vi "HOST_feedback+datatrig_AAoptAOD_8-25-23.vi"() -> ()   [LabVIEW 2020]
uses:
  <vilib>/rvi/interface/nirviMethod/nirviMethod.xnode
  <vilib>/rvi/errors/niLvFpgaMergeErrorWithErrorCode.vi
  <instrlib>/_niInstr/Streaming/v1/Host/niInstr Streaming v1 Host.lvlib
  <vilib>/rvi/interface/nirviReadWriteControl/nirviReadWriteControl.xnode
  <vilib>/rvi/interface/nirviCloseFPGA/nirviCloseFPGA.xnode
  <vilib>/rvi/interface/nirviOpenFPGA/nirviOpenFPGA.xnode
  <vilib>/rvi/interface/Simulation/niFpgaSimulationCallBeginRW.vi
  <vilib>/rvi/errors/niLvFpgaAdjustHostInterfaceError.vi
  NiFpgaLv.dll
  <vilib>/Utility/error.llb/Error Cluster From Error Code.vi
  <vilib>/Utility/file.llb/Write Delimited Spreadsheet (string).vi
  <instrlib>/_niInstr/Streaming/v1/Host/Public/Start Finite Stream.vi
  <instrlib>/_niInstr/Streaming/v1/Host/Public/Wait for Stream.vi
  <vilib>/FPGAPlugInAG/Dynamic/niLvFpga_ConfigureFifo_Dynamic.vi
  <vilib>/FPGAPlugInAG/Dynamic/niLvFpga_StartFifo_Dynamic.vi
  <vilib>/FPGAPlugInAG/Dynamic/niLvFpga_ReadFifo_Dynamic.vi
  <vilib>/FPGAPlugInAG/Dynamic/niLvFpga_WriteFifo_Dynamic.vi
  <vilib>/FPGAPlugInAG/Dynamic/niLvFpga_Close_Dynamic.vi
  <vilib>/measure/NI_MAPro.lvlib
  <instrlib>/_niInstr/Streaming/v1/Host/Public/Start Continuous Stream.vi
  FPGA Bitfiles/rfsignal_FPGATarget_feedbackarray+da_BHXJFx-D6v4.lvbitx
  <vilib>/measure/maspectr.llb/FFT Power Spectrum and PSD for N Chan.vi
  <vilib>/FPGAPlugInAG/PXIe-7972R/niLvFpga_Open_PXIe-7972R.vi
  <vilib>/rvi/interface/common/dynamic/niFpgaDynamicAddResources.vi
  <vilib>/userdefined/Silver/nirio_resource_slv.ctl
  Controls/Clock Select.ctl
  PID/Typedef/niFpgaPID_ManualControl.ctl
  PID/Typedef/niFpgaPID_PIDGains.ctl
  PID/Typedef/niFpgaPID_OutputRange.ctl
  PID/Typedef/niFpgaPID_SetpointWeightings.ctl
  PID/Typedef/niFpgaPID_PIDActions.ctl
panel:
  in  "Save data":bool
  in  "File name":string="Z_3mbar_i"
  in  "Save Path Directory":path=path "D:/Lab Data/test"
  out "SUM PSD":cluster{"f0":dbl, "df":dbl, "magnitude":dbl[]}[](graph)
  out "SUM":waveform(dbl)[](graph)=[{"t0"=timestamp(0 s since 1904-01-01), "dt"=0.0002, "Y"=array[1000 elements]}, {"t0"=timestamp(0 s since 1904-01-01), "dt"=0.0002, "Y"=array[1000 elements]}, {"t0"=timestamp(0 s since 1904-01-01), "dt"=0.0002, "Y"=array[1000 elements]}, {"t0"=timestamp(0 s since 1904-01-01), "dt"=0.0002, "Y"=array[1000 elements]}]
  out "Y PSD":cluster{"f0":dbl, "df":dbl, "magnitude":dbl[]}[](graph)
  out "Y":waveform(dbl)[](graph)=[{"t0"=timestamp(0 s since 1904-01-01), "dt"=0.0002, "Y"=array[1000 elements]}, {"t0"=timestamp(0 s since 1904-01-01), "dt"=0.0002, "Y"=array[1000 elements]}, {"t0"=timestamp(0 s since 1904-01-01), "dt"=0.0002, "Y"=array[1000 elements]}, {"t0"=timestamp(0 s since 1904-01-01), "dt"=0.0002, "Y"=array[1000 elements]}]
  out "X PSD":cluster{"f0":dbl, "df":dbl, "magnitude":dbl[]}[](graph)
  out "X":waveform(dbl)[](graph)=[{"t0"=timestamp(0 s since 1904-01-01), "dt"=0.0002, "Y"=array[1000 elements]}, {"t0"=timestamp(0 s since 1904-01-01), "dt"=0.0002, "Y"=array[1000 elements]}, {"t0"=timestamp(0 s since 1904-01-01), "dt"=0.0002, "Y"=array[1000 elements]}, {"t0"=timestamp(0 s since 1904-01-01), "dt"=0.0002, "Y"=array[1000 elements]}]
  in  "Set Point Initialization":bool
  in  "Feedback scaling y":fxp<+,16,4>
  in  "Gains Y":T1[](array[typedef]) {"filter coefficient" min=0 max=1; "proportional gain" step=0.125}
  in  "Gains X":T1[](array[typedef]) {"filter coefficient" min=0 max=1; "proportional gain" step=0.125}
  in  "Data transfer method":bool
  in  "Downsample":i16=1
  in  "Signal Delay (us)":i32=5
  out "actions":T2
  out "error":sgl
  out "output":sgl
  out "error 2":sgl
  out "error 3":sgl
  out "output 3":sgl
  out "actions 3":T2
  out "output 2":sgl
  out "actions 2":T2
  in  "Gains Z":T1[](array[typedef]) {"filter coefficient" min=0 max=1; "proportional gain" step=0.125}
  in  "setpoint weighting 3":T3={"proportional weighting (1)"=1.0, "derivative weighting (0)"=0.0} {"derivative weighting (0)" min=0 max=1; "proportional weighting (1)" min=0 max=1}
  in  "output range 3":T4={"output high (Inf)"=inf, "output low (-Inf)"=-inf}
  in  "manual control 3":T5
  in  "Z reset? (F)":bool
  in  "setpoint weighting 2":T3={"proportional weighting (1)"=1.0, "derivative weighting (0)"=0.0} {"derivative weighting (0)" min=0 max=1; "proportional weighting (1)" min=0 max=1}
  in  "output range 2":T4={"output high (Inf)"=inf, "output low (-Inf)"=-inf}
  in  "manual control 2":T5
  in  "Y reset? (F)":bool
  in  "Feedback scaling z":fxp<+,16,4>
  in  "Feedback scaling x":fxp<+,16,4>
  in  "Apply feedback":bool
  in  "Data Trigger Level (V)":dbl
  in  "Record Size":u32=1024
  out "AI":waveform(dbl)[](graph)
  in  "Data Trigger When":enum8{"Trigger Above", "Trigger Below"}(ring)
  in  "Trigger Type":enum8{"Immediate", "Data Trigger", "TRIG input"}(ring)
  in  "Direction switch":bool
  in  "Step gain values":dbl
  in  "?":bool
  in  "% of max CH 1":dbl=85.0
  in  "% of max CH 0":dbl=90.0
  in  "setpoint weighting":T3={"proportional weighting (1)"=1.0, "derivative weighting (0)"=0.0} {"derivative weighting (0)" min=0 max=1; "proportional weighting (1)" min=0 max=1}
  in  "output range":T4={"output high (Inf)"=inf, "output low (-Inf)"=-inf}
  in  "manual control":T5
  in  "X reset? (F)":bool
  in  "write time ch0":bool
  in  "Record time for power sweep CH0":bool
  in  "Record time for power sweep CH1":bool
  in  "write time ch1":bool
  in  "save path for power calibration (dialog if empty)":path
  out "time check":u16=16
  in  "Cycles per step":u16=30
  in  "Gain Scan Endpoint (CH1)":dbl[](array[numeric])=[100.0, 100.0, 100.0, 100.0, 100.0, 100.0, 100.0, 100.0, 100.0, 100.0, 100.0, 100.0, 100.0, 100.0, 100.0, 100.0, 100.0, 100.0, 100.0, 100.0, 100.0, 100.0, 100.0, 100.0, 100.0, 100.0, 100.0, 100.0, 100.0, 100.0, 100.0, 100.0, 100.0, 100.0, 100.0, 100.0]
  in  "Gain Scan Endpoint (CH0)":dbl[](array[numeric])=[100.0, 100.0, 100.0, 100.0, 100.0, 100.0, 100.0, 100.0, 100.0, 100.0, 100.0, 100.0, 100.0, 100.0, 100.0, 100.0, 100.0, 100.0, 100.0, 100.0, 100.0, 100.0, 100.0, 100.0, 100.0, 100.0, 100.0, 100.0, 100.0, 100.0, 100.0, 100.0, 100.0, 100.0, 100.0, 100.0]
  in  "Scan End Setpoint (CH1)":dbl[](array[numeric])=[23.0, 24.0, 25.0, 26.0, 27.0, 28.0, 23.0, 24.0, 25.0, 26.0, 27.0, 28.0, 23.0, 24.0, 25.0, 26.0, 27.0, 28.0, 23.0, 24.0, 25.0, 26.0, 27.0, 28.0, 23.0, 24.0, 25.0, 26.0, 27.0, 28.0, 23.0, 24.0, 25.0, 26.0, 27.0, 28.0] format="%#_10f"
  in  "Scan CH1":bool
  in  "Scan CH0":bool
  in  "Fq Scan Endpoint (CH0)":dbl[](array[numeric])=[23.0, 23.0, 23.0, 23.0, 23.0, 23.0, 24.0, 24.0, 24.0, 24.0, 24.0, 24.0, 25.0, 25.0, 25.0, 25.0, 25.0, 25.0, 26.0, 26.0, 26.0, 26.0, 26.0, 26.0, 27.0, 27.0, 27.0, 27.0, 27.0, 27.0, 28.0, 28.0, 28.0, 28.0, 28.0, 28.0] format="%#_10f"
  in  "Gain Scan Step Size % (CH1)":dbl=1.0
  in  "Gain Scan Step Size % (CH0)":dbl=1.0
  in  "Fq Scan Step Size MHz (CH1)":dbl=0.1
  in  "Fq Scan Step Size MHz (CH0)":dbl=0.1
  in  "Input pass through\nmode":enum16{"Wire", "Accum-edge"}(ring)=enum."Accum-edge"
  in  "# of beams":u8=36
  in  "Wave Reader CH 1 (MHz)":dbl[](array[numeric])=[23.0, 24.0, 25.0, 26.0, 27.0, 28.0, 23.0, 24.0, 25.0, 26.0, 27.0, 28.0, 23.0, 24.0, 25.0, 26.0, 27.0, 28.0, 23.0, 24.0, 25.0, 26.0, 27.0, 28.0, 23.0, 24.0, 25.0, 26.0, 27.0, 28.0, 23.0, 24.0, 25.0, 26.0, 27.0, 28.0] format="%#_15f"
  in  "Gain CH 1 (%)":dbl[](array[numeric])=[100.0, 100.0, 100.0, 100.0, 100.0, 100.0, 100.0, 100.0, 100.0, 100.0, 100.0, 100.0, 100.0, 100.0, 100.0, 100.0, 100.0, 100.0, 100.0, 100.0, 100.0, 100.0, 100.0, 100.0, 100.0, 100.0, 100.0, 100.0, 100.0, 100.0, 100.0, 100.0, 100.0, 100.0, 100.0, 100.0]
  in  "Remove transition edges":i32=5
  in  "Time per beam in us":i32=20
  in  "stop":bool
  in  "Gain CH 0 (%)":dbl[](array[numeric])=[100.0, 100.0, 100.0, 100.0, 100.0, 100.0, 100.0, 100.0, 100.0, 100.0, 100.0, 100.0, 100.0, 100.0, 100.0, 100.0, 100.0, 100.0, 100.0, 100.0, 100.0, 100.0, 100.0, 100.0, 100.0, 100.0, 100.0, 100.0, 100.0, 100.0, 100.0, 100.0, 100.0, 100.0, 100.0, 100.0]
  in  "Wave Reader CH 0 (MHz)":dbl[](array[numeric])=[23.0, 23.0, 23.0, 23.0, 23.0, 23.0, 24.0, 24.0, 24.0, 24.0, 24.0, 24.0, 25.0, 25.0, 25.0, 25.0, 25.0, 25.0, 26.0, 26.0, 26.0, 26.0, 26.0, 26.0, 27.0, 27.0, 27.0, 27.0, 27.0, 27.0, 28.0, 28.0, 28.0, 28.0, 28.0, 28.0] format="%#_13f"
  in  "Magnitude Initialization Vpp":dbl[](array[numeric])=[1.0, 1.0] format="%0.2p"
  in  "Frequencies (Hz)":dbl[](array[numeric])=[10000.0, 10000.0] format="%5.0p"
  in  "Signal Type":T6(ring)
  in  "Sampling Info":cluster{"Fs":dbl, "#s":dbl}={"Fs"=163840000.0, "#s"=65536.0} {"Fs" format="%#_5p"}
  out "Error Out":errorcluster
  in  "Update Waveform":bool
  in  "Clock Select":T7 items=["Internal Clock", "Internal Clock w/ Ref via CLK/REF IN", "Internal Clock w/ Ref via Sync Clock", "External Clock via CLK/REF IN"]
  in  "Rate of External Sample Clock (MHz)":u16=100 min=60 max=100 step=1
  in  "RIO Resource":T8="RIO0"
  # "Timeshare sampling doesn't work for 1 beam"
  # "General Feedback Settings"
  # "Time cycle loop processing"
  # "up to 65535"
  # "Don't change"
  # "Waveform Initialization"
  # "Controls the Output of the FPGA\nEach row corresponds to one beam created by the AOD\nCH 0 is Output 0 on the FPGA card and controls the () direction on the AOD; CH 1 is Output 1 on the FPGA card and controls the () direction on the AOD\n\nThe  set frequency is the output of the FPGA, this is then mixed with a 50MHz LO to be in the AOD's bandwidth of 75 +- 15MHz\n\nThe gain is the percentage of the 1Vpp initialized voltage to output. It is in percentage and goes from 0 - 100\n\nIt will play the first n rows of tones, \nwhere n is the \"# of beams\" value."
  # "DO NOT CHANGE"
  # "These allow you to smoothly ramp between frequencies or gain settings for each individual beam.\nThe channels scan independently, but it will simultaneously ramp every fq/gain in the channel to their desired point.\nThey should update to match the main control setting when scanning is not enabled."
  # "X Feedback"
  # "Do not change these values while waiting for scan"
  # "Main control for the tones played on FPGA analog out 0\nSets the base, static frequency to play"
  # "Main control for the tones played on FPGA analog out 1\nSets the base, static frequency to play"
  # "Ch 0 Output Waveforms"
  # "Ch 1 Output Waveforms"
  # "Y Feedback"
  # "Ch0"
  # "Ch1"
  # "Z Feedback"
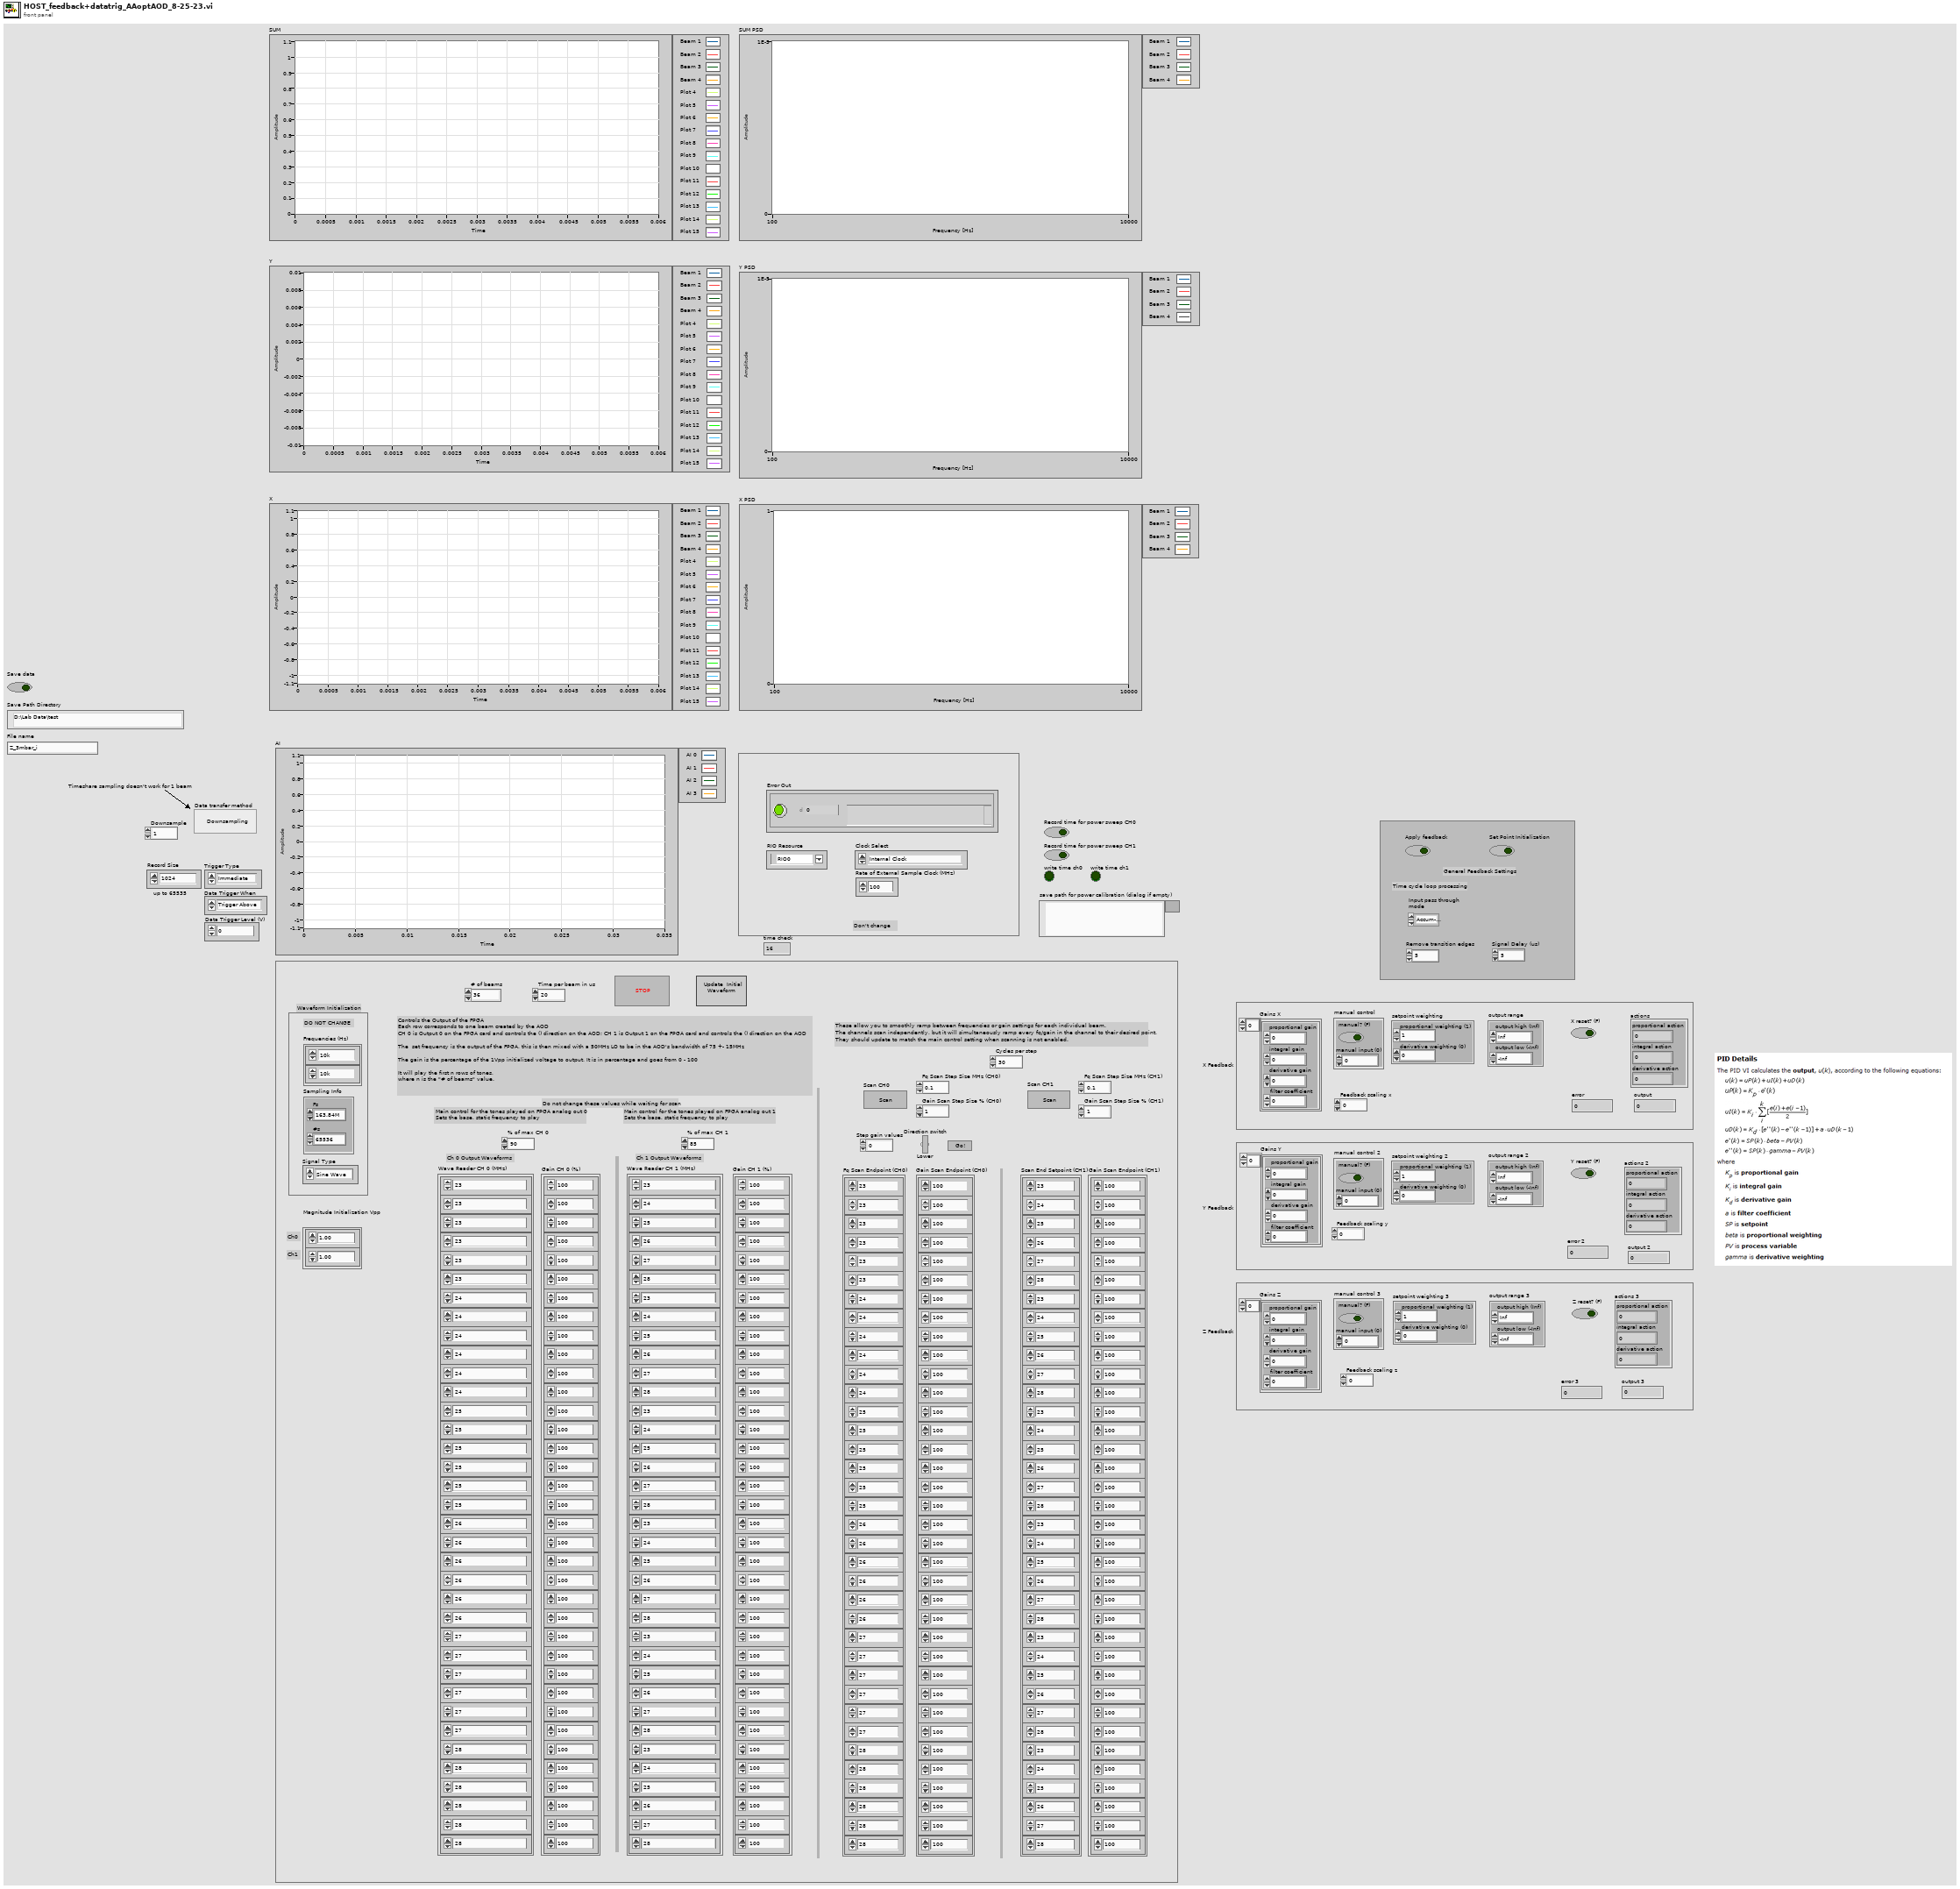
[diagram p1: front panel]
types:
  T1 = typedef "niFpgaPID_PIDGains.ctl" = cluster{"proportional gain":sgl, "integral gain":sgl, "derivative gain":sgl, "filter coefficient":sgl}
  T2 = typedef "niFpgaPID_PIDActions.ctl" = cluster{"proportional action":sgl, "integral action":sgl, "derivative action":sgl}
  T3 = typedef "niFpgaPID_SetpointWeightings.ctl" = cluster{"proportional weighting (1)":sgl, "derivative weighting (0)":sgl}
  T4 = typedef "niFpgaPID_OutputRange.ctl" = cluster{"output high (Inf)":sgl, "output low (-Inf)":sgl}
  T5 = typedef "niFpgaPID_ManualControl.ctl" = cluster{"manual? (F)":bool, "manual input (0)":sgl}
  T6 = enum16{"Sine Wave", "Triangle Wave", "Square Wave", "Sawtooth Wave"}
  T7 = typedef "Clock Select.ctl" = u16
  T8 = typedef "nirio_resource_slv.ctl" = tag
  T9 = cluster{"proportional action":sgl, "integral action":sgl, "derivative action":sgl}
  T10 = cluster{"level":i16, "trigger when":enum8{"Trigger Above", "Trigger Below"}}
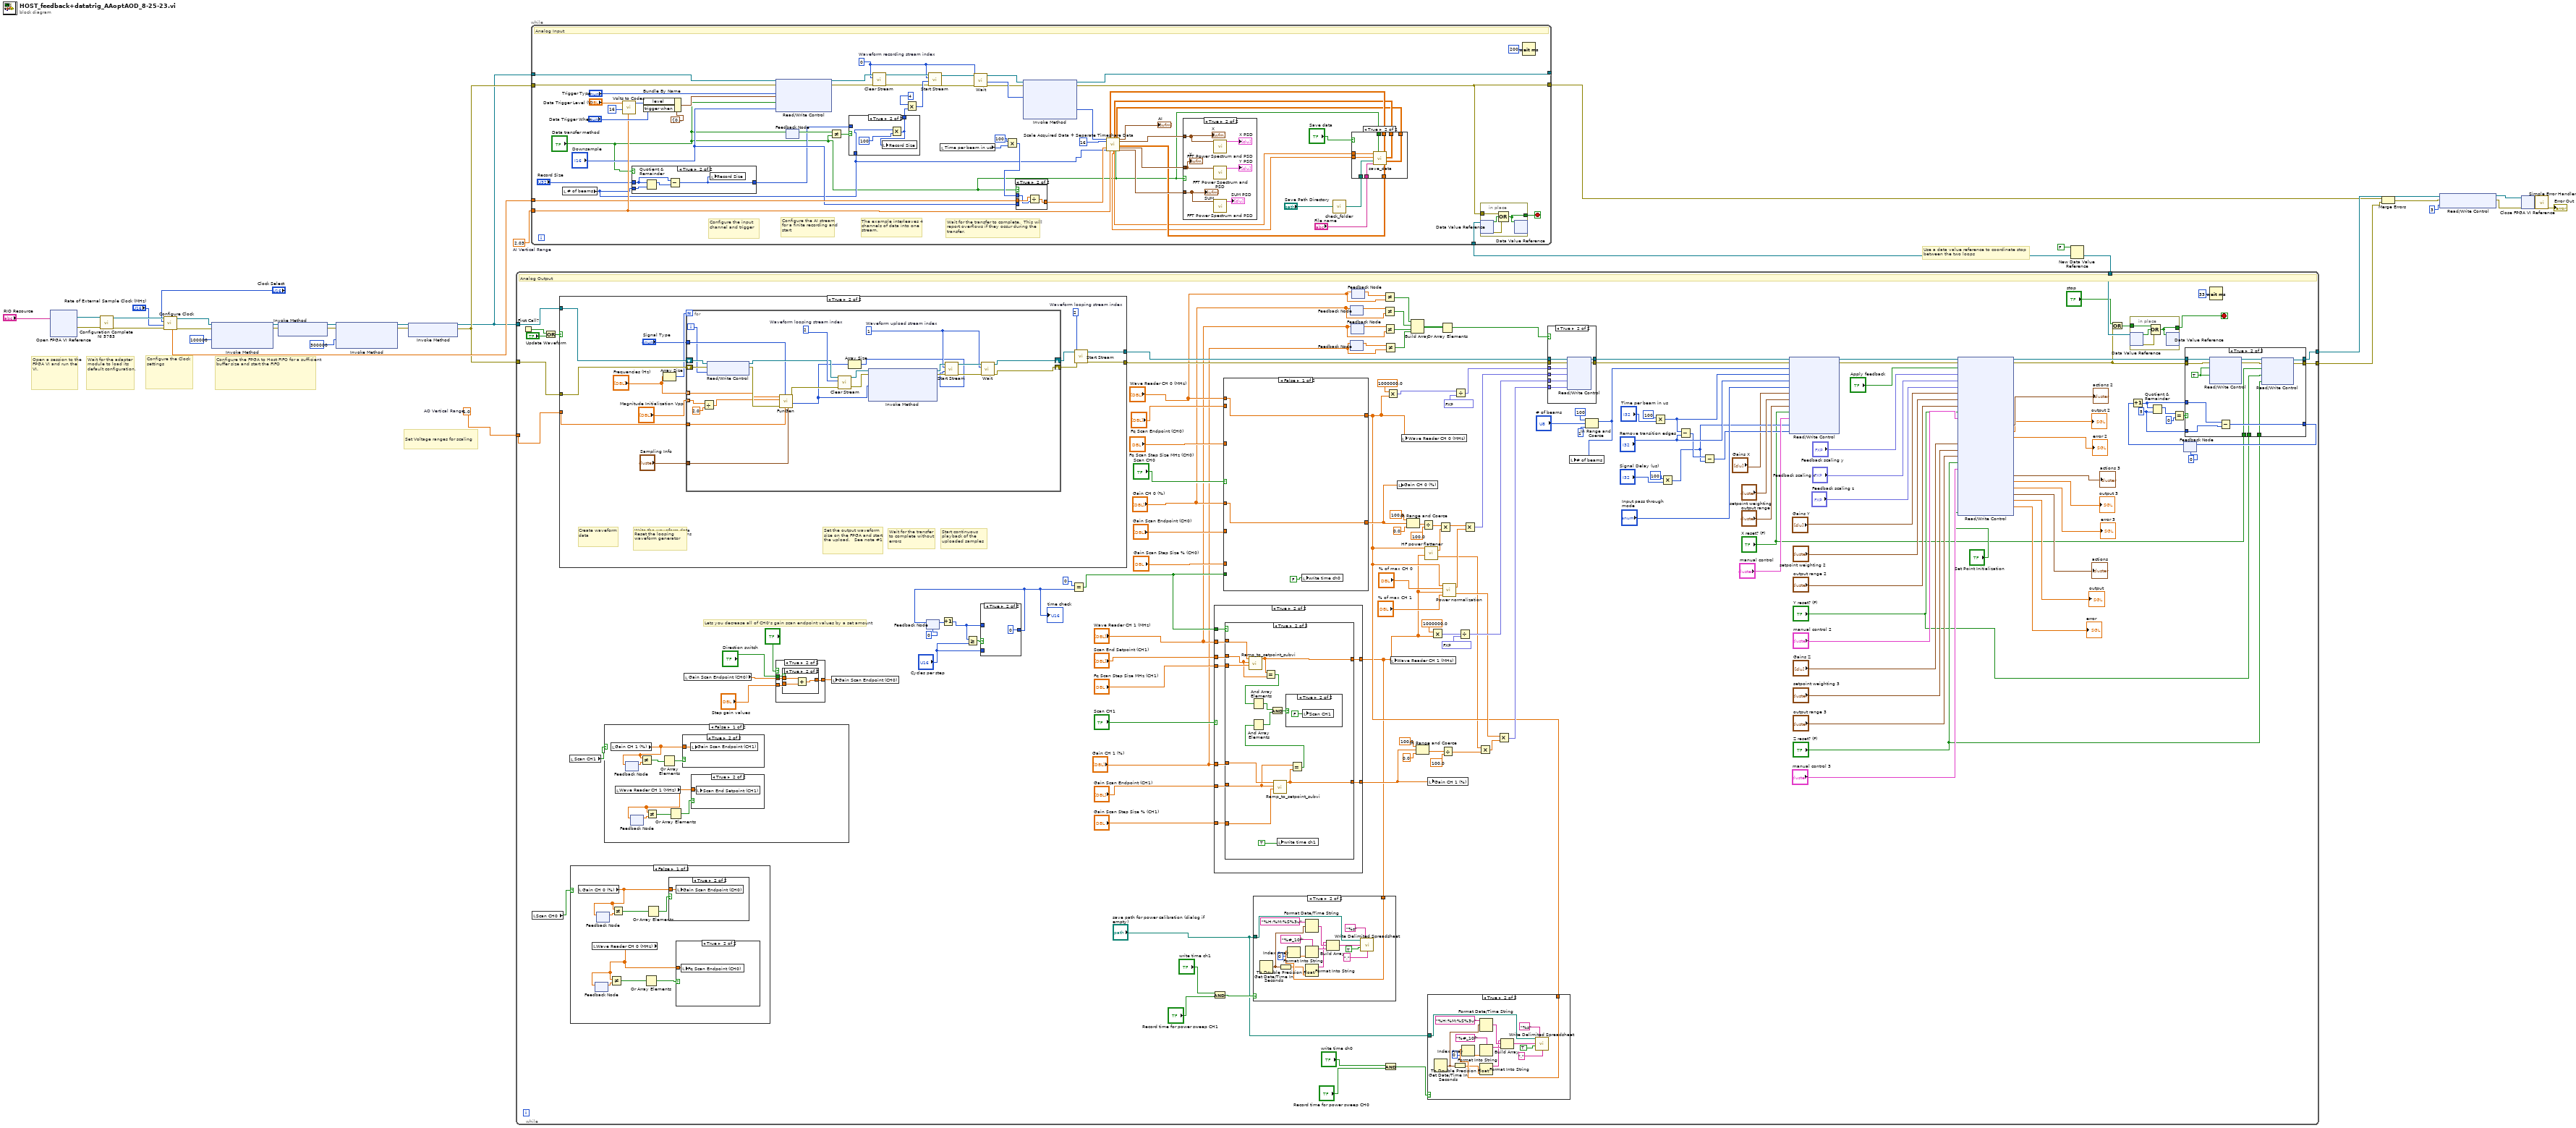
[diagram p0: block diagram]
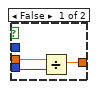
[diagram p6: hidden frame]
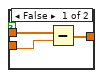
[diagram p10: hidden frame]
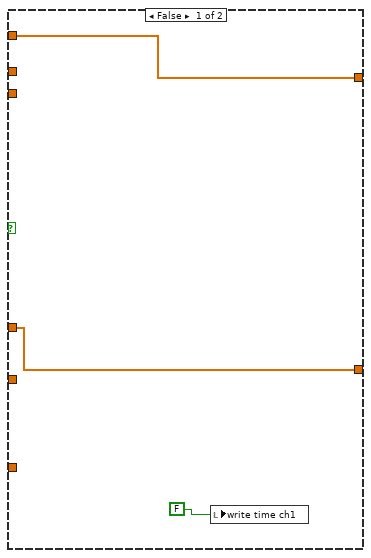
[diagram p13: hidden frame]
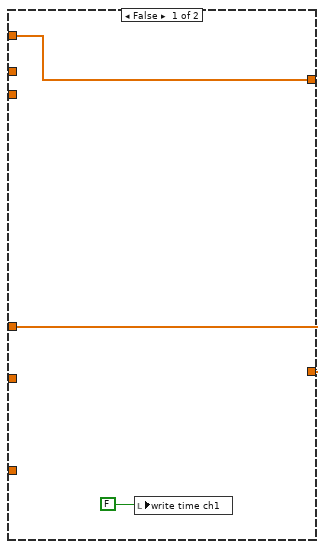
[diagram p14: hidden frame]
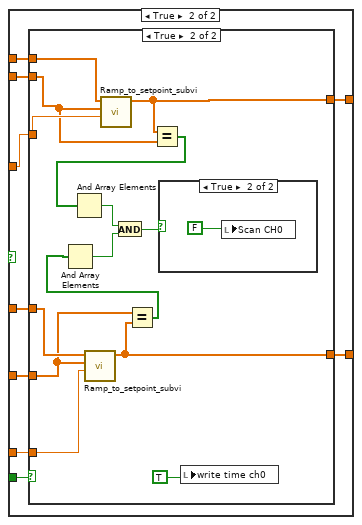
[diagram p16: hidden frame]
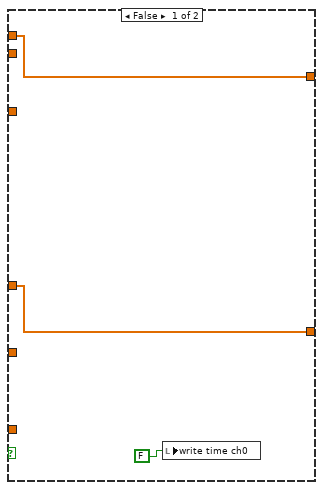
[diagram p17: hidden frame]
diagram:
  w13 = 2.03  # AI Vertical Range
  w21 = 1.0  # AO Vertical Range
  # "Use a data value reference to coordinate stop between the two loops"
  # "Set Voltage ranges for scaling"
  # "Configure the Clock settings"
  # "Configure the FPGA to Host FIFO for a sufficient buffer size and start the FIFO"
  # "Wait for the adapter module to load its default configuration."
  # "Open a session to the FPGA VI and run the VI."
  n1 = xnode "Open FPGA VI Reference"("resource name"="RIO Resource") -> ("FPGA VI Reference Out"=w19:refnum<k20>, "error out"=w18:errorcluster)  [unwired: 1 in]
  n2 = call "Configuration Complete NI 5783.vi"("error in"=w18, "FPGA VI Reference In"=w19) -> ("error out"=w29:errorcluster, "FPGA VI Reference Out"=w30:refnum<k20>)  [unwired: 7 in, 1 out]
  n3 = call "Configure Clock.vi"("error in (no error)"=w29, "Rate of External Sample Clock (MHz)"="Rate of External Sample Clock (MHz)", "Clock Select"="Clock Select", "FPGA VI Reference In"=w30) -> ("error out"=w27:errorcluster, "FPGA VI Reference Out"=w28:refnum<k20>, "Sampling Rate"=w12:dbl)  [unwired: 3 in, 2 out]
  n4 = xnode "Invoke Method"("FPGA VI Reference In"=w28, "error in"=w27, "Requested Depth"=u32 100000) -> ("FPGA VI Reference Out"=w33:refnum<k20>, "error out"=w32:errorcluster)  [unwired: 1 out]
  n5 = xnode "Invoke Method"("FPGA VI Reference In"=w33, "error in"=w32) -> ("FPGA VI Reference Out"=w5:refnum<k20>, "error out"=w8:errorcluster)
  n6 = xnode "Invoke Method"("FPGA VI Reference In"=w5, "error in"=w8, "Requested Depth"=u32 300000) -> ("FPGA VI Reference Out"=w4:refnum<k20>, "error out"=w7:errorcluster)  [unwired: 1 out]
  n7 = xnode "Invoke Method"("FPGA VI Reference In"=w4, "error in"=w7) -> ("FPGA VI Reference Out"=w3:refnum<k20>, "error out"=w6:errorcluster)
  n8 = New Data Value Reference(data value=FALSE ("Stopped")) -> (data value reference=w1:refnum<data-value>)  [unwired: 1 in, 1 out]
  n9 = while {
    tunnel: w6 -> [w177]
    tunnel: w3 -> [w183]
    tunnel: [w39] -> w17
    tunnel: w1 -> [w178]
    tunnel: w21 -> [w176]
    tunnel: [w38] -> w9
    stop <- w108 stop-if-true
    w41 = 5
    # "Lets you decrease all of CH0's gain scan endpoint values by a set amount"
    # "Analog Output"
    n10 = First Call?() -> (First Call?: T/F=w179:bool)
    n11 = local read "Scan CH0"() -> (w146:bool)
    n12 = Or(x=w179, y="Update Waveform") -> (x .or. y?=w180:bool)
    n13 = case shown="True" w180 {
      tunnel: [w338 w351] -> w175
      tunnel: [w337 w350] -> w174
      tunnel: w183 -> [w338 w348]
      tunnel: w177 -> [w337 w347]
      tunnel: w176 -> [_ w349]
      frame False {
      }
      frame True {
        w346 = 2  # Waveform looping stream index
        # "Loop over the waveforms to combine"
        # "Reset the looping waveform generator"
        # "Start continuous playback of the uploaded samples"
        # "Wait for the transfer to complete without errors"
        # "Set the output waveform size on the FPGA and start the upload.   See note #1"
        # "Write the waveform data to the FPGA for generation"
        # "Create waveform data"
        n14 = Array Size(array="Frequencies (Hz)") -> (size(s)=w341:i32)
        n15 = for {
          N: w341 -> [_]
          tunnel: w349 -> [w366]
          shift-right: [w360] -> w345
          shift-left: w348 -> [w365]
          shift-right: [w359] -> w344
          shift-left: w347 -> [w363]
          tunnel: "Frequencies (Hz)" -> [w358] mode=indexing
          tunnel: "Magnitude Initialization Vpp" -> [w354] mode=indexing
          tunnel: "Sampling Info" -> [w357]
          tunnel: "Signal Type" -> [w356]
          i -> [w355]
          w367 = 2  # Waveform looping stream index
          w372 = 1  # Waveform upload stream index
          n16 = Divide(x=w354, y=2.0) -> (x/y=w353:dbl)
          n17 = xnode "Read/Write Control"("FPGA VI Reference In"=w365, "error in"=w363, "Upload selector"=w355) -> ("FPGA VI Reference Out"=w364:refnum<k20>, "error out"=w362:errorcluster)
          n18 = call "FunGen.vi"("sampling info"=w357, "range (Vpp)"=w366, "signal type"=w356, "error in (no error)"=w362, "amplitude"=w353, "frequency"=w358) -> ("error out"=w368:errorcluster, "Waveform Data"=w361:i16[])  [unwired: 2 in, 2 out]
          n19 = call <instrlib>:"Clear Stream.vi"("error in (no error)"=w368, "stream index"=w367, "refnum in"=w364) -> ("error out"=w370:errorcluster, "refnum out"=w371:refnum<k20>)  [unwired: 7 in]
          n20 = Array Size(array=w361) -> (size(s)=w369:i32)
          n21 = xnode "Invoke Method"("FPGA VI Reference In"=w371, "error in"=w370, "Data"=w361) -> ("FPGA VI Reference Out"=w376:refnum<k20>, "error out"=w375:errorcluster)  [unwired: 1 in, 1 out]
          n22 = call-poly <instrlib>:"Start Stream.vi"("error in (no error)"=w375, "num samples"=w369, "stream index"=w372, "refnum in"=w376) -> ("error out"=w373:errorcluster, "refnum out"=w374:refnum<k20>)  [unwired: 6 in]
          n23 = call-poly <instrlib>:"Wait.vi"("error in (no error)"=w373, "stream index"=w372, "refnum in"=w374) -> ("error out"=w359:errorcluster, "refnum out"=w360:refnum<k20>)  [unwired: 5 in, 2 out]
        }
        n24 = call-poly <instrlib>:"Start Stream.vi"("error in (no error)"=w344, "stream index"=w346, "refnum in"=w345) -> ("error out"=w350:errorcluster, "refnum out"=w351:refnum<k20>)  [unwired: 7 in]
      }
    }
    n25 = local read "Scan CH1"() -> (w147:bool)
    n26 = case shown="False" w146 {
      frame False {
        n27 = local read "Gain CH 0 (%)"() -> (w313:dbl[])
        n28 = local read "Wave Reader CH 0 (MHz)"() -> (w320:dbl[])
        n29 = feedback-in #1(w320) -> ()
        n30 = feedback #1() -> (w319:dbl[])  [unwired: 1 in]
        n31 = feedback #2() -> (w316:dbl[])  [unwired: 1 in]
        n32 = feedback-in #2(w313) -> ()
        n33 = Not Equal?(x=w320, y=w319) -> (x != y?=w318:bool[])
        n34 = Not Equal?(x=w313, y=w316) -> (x != y?=w315:bool[])
        n35 = Or Array Elements(Boolean array=w318) -> (logical OR=w317:bool)
        n36 = Or Array Elements(Boolean array=w315) -> (logical OR=w314:bool)
        n37 = case shown="True" w314 {
          tunnel: w313 -> [_ w321]
          frame False {
          }
          frame True {
            n38 = local write "Gain Scan Endpoint (CH0)"(w321) -> ()
          }
        }
        n39 = case shown="True" w317 {
          tunnel: w320 -> [_ w322]
          frame False {
          }
          frame True {
            n40 = local write "Fq Scan Endpoint (CH0)"(w322) -> ()
          }
        }
      }
      frame True {
      }
    }
    n41 = case shown="False" w147 {
      frame False {
        n42 = local read "Gain CH 1 (%)"() -> (w323:dbl[])
        n43 = local read "Wave Reader CH 1 (MHz)"() -> (w327:dbl[])
        n44 = feedback #3() -> (w326:dbl[])  [unwired: 1 in]
        n45 = feedback-in #3(w323) -> ()
        n46 = feedback #4() -> (w330:dbl[])  [unwired: 1 in]
        n47 = feedback-in #4(w327) -> ()
        n48 = Not Equal?(x=w323, y=w326) -> (x != y?=w325:bool[])
        n49 = Not Equal?(x=w327, y=w330) -> (x != y?=w329:bool[])
        n50 = Or Array Elements(Boolean array=w325) -> (logical OR=w324:bool)
        n51 = Or Array Elements(Boolean array=w329) -> (logical OR=w328:bool)
        n52 = case shown="True" w324 {
          tunnel: w323 -> [_ w331]
          frame False {
          }
          frame True {
            n53 = local write "Gain Scan Endpoint (CH1)"(w331) -> ()
          }
        }
        n54 = case shown="True" w328 {
          tunnel: w327 -> [_ w332]
          frame False {
          }
          frame True {
            n55 = local write "Scan End Setpoint (CH1)"(w332) -> ()
          }
        }
      }
      frame True {
      }
    }
    n56 = local read "Gain Scan Endpoint (CH0)"() -> (w110:dbl[])
    n57 = case shown="True" "?" {
      tunnel: w110 -> [w210 w213]
      tunnel: [w210 w214] -> w111
      tunnel: "Step gain values" -> [_ w212]
      tunnel: "Direction switch" -> [_ w211]
      frame False {
      }
      frame True {
        n58 = case shown="True" w211 {
          tunnel: [w217 w219] -> w214
          tunnel: w213 -> [w216 w218]
          tunnel: w212 -> [w215 w220]
          frame False {
            n59 = Subtract(x=w216, y=w215) -> (x-y=w217:dbl[])
          }
          frame True {
            n60 = Add(x=w218, y=w220) -> (x+y=w219:dbl[])
          }
        }
      }
    }
    n61 = local write "Gain Scan Endpoint (CH0)"(w111) -> ()
    n62 = feedback #5(u16 0) -> (w142:u16)
    n63 = Increment(x=w142) -> (x+1=w140:u16)
    n64 = Greater Or Equal?(x=w140, y="Cycles per step") -> (x >= y?=w141:bool)
    n65 = case shown="True" w141 {
      tunnel: w140 -> [w311 _]
      tunnel: "Cycles per step" -> [_ _]
      tunnel: [w311 u16 0] -> w135
      frame False {
      }
      frame True {
      }
    }
    "time check" <- w135
    n66 = feedback-in #5(w135) -> ()
    n67 = Equal?(x=u16 0, y=w135) -> (x = y?=w136:bool)
    n68 = And(x="write time ch1", y="Record time for power sweep CH1") -> (x .and. y?=w134:bool)
    n69 = case shown="True" "Scan CH1" {
      tunnel: "Fq Scan Step Size MHz (CH1)" -> [_ w262]
      tunnel: [w253 w261] -> w70
      tunnel: "Wave Reader CH 1 (MHz)" -> [w253 w260]
      tunnel: "Scan End Setpoint (CH1)" -> [_ w259]
      tunnel: "Gain Scan Step Size % (CH1)" -> [_ w258]
      tunnel: "Gain CH 1 (%)" -> [w252 w257]
      tunnel: "Gain Scan Endpoint (CH1)" -> [_ w256]
      tunnel: [w252 w255] -> w148
      tunnel: w136 -> [_ w254]
      frame False {
        n70 = local write "write time ch1"(FALSE) -> ()
      }
      frame True {
        n71 = case shown="True" w254 {
          tunnel: w260 -> [w265 w279]
          tunnel: w259 -> [_ w277]
          tunnel: w262 -> [_ w278]
          tunnel: [w265 w276] -> w261
          tunnel: w257 -> [w264 w274]
          tunnel: w256 -> [_ w273]
          tunnel: w258 -> [_ w272]
          tunnel: [w264 w267] -> w255
          frame False {
            n72 = local write "write time ch1"(FALSE) -> ()
          }
          frame True {
            n73 = call "Ramp_to_setpoint_subvi.vi"("Numeric"=w278, "Scan to Fq (CH0)"=w277, "Wave Reader CH 0 (Y)"=w279) -> ("Array"=w276:dbl[])  [unwired: 8 in]
            n74 = Equal?(x=w276, y=w277) -> (x = y?=w275:bool[])
            n75 = And Array Elements(Boolean array=w275) -> (logical AND=w269:bool)
            n76 = call "Ramp_to_setpoint_subvi.vi"("Numeric"=w272, "Scan to Fq (CH0)"=w273, "Wave Reader CH 0 (Y)"=w274) -> ("Array"=w267:dbl[])  [unwired: 8 in]
            n77 = local write "write time ch1"(TRUE) -> ()
            n78 = Equal?(x=w273, y=w267) -> (x = y?=w268:bool[])
            n79 = And Array Elements(Boolean array=w268) -> (logical AND=w270:bool)
            n80 = And(x=w269, y=w270) -> (x .and. y?=w271:bool)
            n81 = case shown="True" w271 {
              frame False {
              }
              frame True {
                n82 = local write "Scan CH1"(FALSE) -> ()
              }
            }
          }
        }
      }
    }
    n83 = case shown="False" "Scan CH0" {
      tunnel: "Fq Scan Step Size MHz (CH0)" -> [_ w292]
      tunnel: "Wave Reader CH 0 (MHz)" -> [w283 w291]
      tunnel: "Fq Scan Endpoint (CH0)" -> [_ w290]
      tunnel: [w283 w289] -> w73
      tunnel: "Gain CH 0 (%)" -> [w282 w288]
      tunnel: "Gain Scan Endpoint (CH0)" -> [_ w287]
      tunnel: [w282 w286] -> w155
      tunnel: "Gain Scan Step Size % (CH0)" -> [_ w285]
      tunnel: w136 -> [_ w284]
      frame False {
        n84 = local write "write time ch0"(FALSE) -> ()
      }
      frame True {
        n85 = case shown="True" w284 {
          tunnel: w291 -> [w295 w309]
          tunnel: w290 -> [_ w307]
          tunnel: w292 -> [_ w308]
          tunnel: [w295 w306] -> w289
          tunnel: w288 -> [w294 w304]
          tunnel: w287 -> [_ w301]
          tunnel: w285 -> [_ w303]
          tunnel: [w294 w302] -> w286
          frame False {
            n86 = local write "write time ch0"(FALSE) -> ()
          }
          frame True {
            n87 = call "Ramp_to_setpoint_subvi.vi"("Numeric"=w303, "Scan to Fq (CH0)"=w301, "Wave Reader CH 0 (Y)"=w304) -> ("Array"=w302:dbl[])  [unwired: 8 in]
            n88 = call "Ramp_to_setpoint_subvi.vi"("Numeric"=w308, "Scan to Fq (CH0)"=w307, "Wave Reader CH 0 (Y)"=w309) -> ("Array"=w306:dbl[])  [unwired: 8 in]
            n89 = Equal?(x=w301, y=w302) -> (x = y?=w300:bool[])
            n90 = And Array Elements(Boolean array=w300) -> (logical AND=w297:bool)
            n91 = Equal?(x=w306, y=w307) -> (x = y?=w305:bool[])
            n92 = And Array Elements(Boolean array=w305) -> (logical AND=w298:bool)
            n93 = And(x=w298, y=w297) -> (x .and. y?=w299:bool)
            n94 = case shown="True" w299 {
              frame False {
              }
              frame True {
                n95 = local write "Scan CH0"(FALSE) -> ()
              }
            }
            n96 = local write "write time ch0"(TRUE) -> ()
          }
        }
      }
    }
    n97 = case shown="True" w134 {
      tunnel: w70 -> [_ w243]
      tunnel: "save path for power calibration (dialog if empty)" -> [_ w236]
      frame False {
      }
      frame True {
        n98 = Get Date/Time In Seconds() -> (seconds since 1Jan1904=w239:timestamp)
        n99 = To Double Precision Float(number=w239) -> (double precision float=w238:dbl)
        n100 = Index Array(array=w243, index=0) -> (element=w241:dbl)
        n101 = Format Date/Time String(time format string (%c)="%H:%M:%S%3u", seconds (now)=w239) -> (date/time string=w246:string)  [unwired: 1 in]
        n102 = Format Into String(format string="%#_10f", w241) -> (resulting string=w245:string)  [unwired: 2 in, 1 out]
        n103 = Format Into String(w238) -> (resulting string=w237:string)  [unwired: 3 in, 1 out]
        n104 = Build Array(w237, w246, w245) -> (w240:string[])
        n105 = call-poly <vilib>:"Write Delimited Spreadsheet.vi"("file path (dialog if empty)"=w236, "format (%s)"="%s" ("format (%.3f)"), "1D data"=w240, "append to file? (new file:F)"=TRUE, "delimiter (\\t)"="," ("delimiter (\\t)")) -> ()  [unwired: 9 in, 2 out]
      }
    }
    n106 = feedback-in #6("Gain CH 0 (%)") -> ()
    n107 = feedback #6() -> (w64:dbl[])  [unwired: 1 in]
    n108 = feedback #7() -> (w60:dbl[])  [unwired: 1 in]
    n109 = feedback-in #7("Gain CH 1 (%)") -> ()
    n110 = feedback #8() -> (w62:dbl[])  [unwired: 1 in]
    n111 = feedback-in #8("Wave Reader CH 1 (MHz)") -> ()
    n112 = feedback #9() -> (w65:dbl[])  [unwired: 1 in]
    n113 = feedback-in #9("Wave Reader CH 0 (MHz)") -> ()
    n114 = Not Equal?(x=w65, y="Wave Reader CH 0 (MHz)") -> (x != y?=w58:bool[])
    n115 = Not Equal?(x=w64, y="Gain CH 0 (%)") -> (x != y?=w57:bool[])
    n116 = Not Equal?(x=w62, y="Wave Reader CH 1 (MHz)") -> (x != y?=w56:bool[])
    n117 = Not Equal?(x=w60, y="Gain CH 1 (%)") -> (x != y?=w55:bool[])
    n118 = And(x="write time ch0", y="Record time for power sweep CH0") -> (x .and. y?=w130:bool)
    n119 = Multiply(x=1000000.0, y=w73) -> (x*y=w164:fxp<+/-,64,32>[])
    n120 = local write "Wave Reader CH 1 (MHz)"(w70) -> ()
    n121 = local write "Gain CH 0 (%)"(w155) -> ()
    n122 = local write "Wave Reader CH 0 (MHz)"(w73) -> ()
    n123 = In Range and Coerce(upper limit=100.0, x=w155, lower limit=0.0) -> (coerced(x)=w158:dbl[])  [unwired: 1 out]
    n124 = Build Array(w58, w57, w56, w55) -> (w54:bool[][])
    n125 = In Range and Coerce(upper limit=100.0, x=w148, lower limit=0.0) -> (coerced(x)=w153:dbl[])  [unwired: 1 out]
    n126 = Divide(x=w158, y=100.0) -> (x/y=w121:dbl[])
    n127 = call "HF power flattener.vi"("CH 1 frequency"=w70, "CH 0 frequency"=w73) -> ("Normalized CH1"=w67:dbl[], "Normalized CH 0"=w71:dbl[])  [unwired: 2 in]
    n128 = local write "Gain CH 1 (%)"(w148) -> ()
    n129 = case shown="True" w130 {
      tunnel: w73 -> [_ w228]
      tunnel: "save path for power calibration (dialog if empty)" -> [_ w221]
      frame False {
      }
      frame True {
        n130 = Get Date/Time In Seconds() -> (seconds since 1Jan1904=w224:timestamp)
        n131 = To Double Precision Float(number=w224) -> (double precision float=w223:dbl)
        n132 = Index Array(array=w228, index=0) -> (element=w226:dbl)
        n133 = Format Date/Time String(time format string (%c)="%H:%M:%S%3u", seconds (now)=w224) -> (date/time string=w231:string)  [unwired: 1 in]
        n134 = Format Into String(format string="%#_10f", w226) -> (resulting string=w230:string)  [unwired: 2 in, 1 out]
        n135 = Format Into String(w223) -> (resulting string=w222:string)  [unwired: 3 in, 1 out]
        n136 = Build Array(w222, w231, w230) -> (w225:string[])
        n137 = call-poly <vilib>:"Write Delimited Spreadsheet.vi"("file path (dialog if empty)"=w221, "format (%s)"="%s" ("format (%.3f)"), "1D data"=w225, "append to file? (new file:F)"=TRUE, "delimiter (\\t)"="," ("delimiter (\\t)")) -> ()  [unwired: 9 in, 2 out]
      }
    }
    n138 = Multiply(x=1000000.0, y=w70) -> (x*y=w162:fxp<+/-,64,32>[])
    n139 = Multiply(x=w121, y=w71) -> (x*y=w72:dbl[])
    n140 = Or Array Elements(Boolean array=w54) -> (logical OR=w53:bool)
    n141 = Divide(x=w153, y=100.0) -> (x/y=w68:dbl[])
    n142 = call "Power normalization.vi"("% of max CH 1"="% of max CH 1", "CH 1 frequency"=w70, "% of max CH 0"="% of max CH 0", "CH 0 frequency"=w73) -> ("Normalized CH1"=w116:dbl[], "Normalized CH 0"=w118:dbl[])
    n143 = Divide(x=w164, y=fxp<+,32,16> 6103.515625) -> (x/y=w127:fxp<+,33,16>[])
    n144 = Divide(x=w162, y=fxp<+,32,16> 6103.515625) -> (x/y=w126:fxp<+,33,16>[])
    n145 = Multiply(x=w72, y=w118) -> (x*y=w122:fxp<+,32,4>[])
    n146 = Multiply(x=w67, y=w68) -> (x*y=w69:dbl[])
    n147 = Multiply(x=w116, y=w69) -> (x*y=w117:fxp<+,32,4>[])
    n148 = case shown="True" w53 {
      tunnel: w175 -> [w201 w209]
      tunnel: w174 -> [w200 w208]
      tunnel: [w201 w207] -> w172
      tunnel: [w200 w206] -> w171
      tunnel: w127 -> [_ w205]
      tunnel: w126 -> [_ w204]
      tunnel: w122 -> [_ w203]
      tunnel: w117 -> [_ w202]
      frame False {
      }
      frame True {
        n149 = xnode "Read/Write Control"("FPGA VI Reference In"=w209, "error in"=w208, "Wave 1"=w205, "Amp 1"=w203, "Wave 2"=w204, "Amp 2"=w202) -> ("FPGA VI Reference Out"=w207:refnum<k20>, "error out"=w206:errorcluster)
      }
    }
    n150 = In Range and Coerce(upper limit=u8 100, x="# of beams", lower limit=u8 1) -> (coerced(x)=w49:u8)  [unwired: 1 out]
    n151 = local write "# of beams"(w49) -> ()
    n152 = Multiply(x=100, y="Time per beam in us") -> (x*y=w85:i32)
    n153 = Multiply(x=100, y="Signal Delay (us)") -> (x*y=w82:i32)
    n154 = Subtract(x=w85, y="Remove transition edges") -> (x-y=w83:i32)
    n155 = Subtract(x=w83, y=w82) -> (x-y=w81:i32)
    n156 = xnode "Read/Write Control"("FPGA VI Reference In"=w172, "error in"=w171, "Size"=w49, "Timeshare"=w85, "Edge size"="Remove transition edges", "Pass selector"="Input pass through\nmode", "Gains X"="Gains X", "setpoint weighting"="setpoint weighting", "output range"="output range", "X reset? (F)"="X reset? (F)", "manual control"="manual control", "Signal Delay"=w82, "Data collection size"=w81) -> ("FPGA VI Reference Out"=w104:refnum<k20>, "error out"=w105:errorcluster)
    n157 = xnode "Read/Write Control"("FPGA VI Reference In"=w104, "error in"=w105, "Apply feedback"="Apply feedback", "Feedback scaling y"="Feedback scaling y", "Feedback scaling x"="Feedback scaling x", "Feedback scaling z"="Feedback scaling z", "Gains Y"="Gains Y", "setpoint weighting 2"="setpoint weighting 2", "output range 2"="output range 2", "Y reset? (F)"="Y reset? (F)", "manual control 2"="manual control 2", "Gains Z"="Gains Z", "setpoint weighting 3"="setpoint weighting 3", "output range 3"="output range 3", "Z reset? (F)"="Z reset? (F)", "manual control 3"="manual control 3", "Set Point Initialization"="Set Point Initialization") -> ("FPGA VI Reference Out"=w40:refnum<k20>, "error out"=w37:errorcluster, "actions 2"=→"actions 2":T9, "output 2"=→"output 2":sgl, "error 2"=→"error 2":sgl, "actions 3"=→"actions 3":T9, "output 3"=→"output 3":sgl, "error 3"=→"error 3":sgl, "actions"=→"actions":T9, "output"=→"output":sgl, "error"=→"error":sgl)
    n158 = Or(x="stop", y=w37) -> (x .or. y?=w107:bool)
    n159 = in-place {
      in-place-border: [w335] -> w108
      in-place-border: w107 -> [w333]
      n160 = in-place-dvr #10(w178) -> (w336:bool, w334:errorcluster)
      n161 = Compound Arithmetic op=OR(w333, w336, w334) -> (w335:bool)
      n162 = in-place-dvr #10(w335) -> ()  [unwired: 2 out]
    }
    n163 = feedback #11(0) -> (w47:i32)
    n164 = Increment(x=w47) -> (x+1=w45:i32)
    n165 = Quotient & Remainder(x=w45, y=w41) -> (x-y*floor(x/y)=w43:i32)  [unwired: 1 out]
    n166 = Equal?(x=w43, y=0) -> (x = y?=w44:bool)
    n167 = case shown="True" w44 {
      tunnel: [w184 w198] -> w48
      tunnel: w45 -> [w184 w199]
      tunnel: w41 -> [_ w197]
      tunnel: w40 -> [w186 w196]
      tunnel: [w186 w190] -> w39
      tunnel: [w185 w191] -> w38
      tunnel: w37 -> [w185 w195]
      tunnel: "Z reset? (F)" -> [_ w189]
      tunnel: "Y reset? (F)" -> [_ w188]
      tunnel: "X reset? (F)" -> [_ w187]
      frame False {
      }
      frame True {
        w194 = TRUE
        n168 = xnode "Read/Write Control"("FPGA VI Reference In"=w196, "error in"=w195, "X reset? (F)"=w194, "Y reset? (F)"=w194, "Z reset? (F)"=w194) -> ("FPGA VI Reference Out"=w193:refnum<k20>, "error out"=w192:errorcluster)
        n169 = Subtract(x=w199, y=w197) -> (x-y=w198:i32)
        n170 = xnode "Read/Write Control"("FPGA VI Reference In"=w193, "error in"=w192, "X reset? (F)"=w187, "Y reset? (F)"=w188, "Z reset? (F)"=w189) -> ("FPGA VI Reference Out"=w190:refnum<k20>, "error out"=w191:errorcluster)
      }
    }
    n171 = feedback-in #11(w48) -> ()
    n172 = Wait (ms)(milliseconds to wait=u32 33) -> ()  [unwired: 1 out]
  }
  n173 = while {
    tunnel: [w431] -> _
    tunnel: w3 -> [w430]
    tunnel: w13 -> [w414]
    tunnel: w1 -> [w427]
    tunnel: w6 -> [w429]
    tunnel: [w418] -> w10
    tunnel: w12 -> [w404]
    stop <- w428 stop-if-true
    w408 = 0  # Waveform recording stream index
    # "The example interleaves 4 channels of data into one stream."
    # "Wait for the transfer to complete.  This will report overflows if they occur during the transfer."
    # "Configure the AI stream for a finite recording and start"
    # "Configure the input channel and trigger"
    # "Analog Input"
    n174 = local read "# of beams"() -> (w379:u8)
    n175 = call "Volts to Codes.vi"("range (Vpp)"=w414, "Number of Bits"=i16 16, "Volts In"="Data Trigger Level (V)") -> ("ADC Codes Out"=w415:i16)  [unwired: 8 in]
    n176 = case shown="True" "Data transfer method" {
      tunnel: "Record Size" -> [w442 w445]
      tunnel: [w442 w443] -> w393
      tunnel: w379 -> [_ w446]
      frame False {
      }
      frame True {
        n177 = Quotient & Remainder(x=w445, y=w446) -> (x-y*floor(x/y)=w444:u32)  [unwired: 1 out]
        n178 = Subtract(x=w445, y=w444) -> (x-y=w443:u32)
        n179 = local write "Record Size"(w443) -> ()
      }
    }
    n180 = Bundle By Name(cluster=T10 {"level"=0, "trigger when"=enum."Trigger Above"} ("Trigger Configuration"), "level"=w415, "trigger when"="Data Trigger When") -> (w407:T10)
    n181 = xnode "Read/Write Control"("FPGA VI Reference In"=w430, "error in"=w429, "Trigger Type"="Trigger Type", "Trigger Configuration"=w407, "Data transfer method"="Data transfer method", "Downsample"="Downsample") -> ("FPGA VI Reference Out"=w412:refnum<k20>, "error out"=w411:errorcluster)
    n182 = feedback-in #12("Data transfer method") -> ()
    n183 = feedback #12() -> (w394:bool)  [unwired: 1 in]
    n184 = Not Equal?(x=w394, y="Data transfer method") -> (x != y?=w395:bool)
    n185 = case shown="True" w395 {
      tunnel: w393 -> [w447 _]
      tunnel: [w447 w450] -> w392
      tunnel: w379 -> [_ w448]
      frame False {
      }
      frame True {
        n186 = Multiply(x=w448, y=100) -> (x*y=w450:u32)
        n187 = local write "Record Size"(w450) -> ()
      }
    }
    n188 = call <instrlib>:"Clear Stream.vi"("error in (no error)"=w411, "stream index"=w408, "refnum in"=w412) -> ("error out"=w410:errorcluster, "refnum out"=w409:refnum<k20>)  [unwired: 7 in]
    n189 = Multiply(x=u16 4 ("y"), y=w392) -> (x*y=w413:u32)
    n190 = call-poly <instrlib>:"Start Stream.vi"("error in (no error)"=w410, "num samples"=w413, "stream index"=w408, "refnum in"=w409) -> ("error out"=w423:errorcluster, "refnum out"=w421:refnum<k20>)  [unwired: 6 in]
    n191 = local read "Time per beam in us"() -> (w400:i32)
    n192 = call-poly <instrlib>:"Wait.vi"("error in (no error)"=w423, "stream index"=w408, "refnum in"=w421) -> ("error out"=w419:errorcluster, "samples transferred"=w422:u64, "refnum out"=w420:refnum<k20>)  [unwired: 5 in, 1 out]
    n193 = Multiply(x=100, y=w400) -> (x*y=w390:i32)
    n194 = case shown="True" "Data transfer method" {
      tunnel: w404 -> [w459 w462]
      tunnel: [w458 w460] -> w403
      tunnel: "Downsample" -> [w457 _]
      tunnel: w390 -> [_ w461]
      frame False {
        n195 = Divide(x=w459, y=w457) -> (x/y=w458:dbl)
      }
      frame True {
        n196 = Divide(x=w462, y=w461) -> (x/y=w460:dbl)
      }
    }
    n197 = xnode "Invoke Method"("FPGA VI Reference In"=w420, "error in"=w419, "Number of Elements"=w422) -> ("FPGA VI Reference Out"=w431:refnum<k20>, "error out"=w418:errorcluster, "Data"=w399:i16[])  [unwired: 1 in, 1 out]
    n198 = call "Scale Acquired Data + Separate Timeshare Data.vi"("Data In"=w399, "Number of Bits"=i16 16, "Sample Rate"=w403, "Array size"=w379, "range (V)"=w414, "Timeshare sampling"="Data transfer method") -> ("Beam sorted X data"=w386:dbl[][], "AI stream sampling rate"=w381:dbl, "Beam sorted Y data"=w385:dbl[][], "Beam sorted sampling rate"=w382:dbl, "Beam sorted SUM data"=w384:dbl[][], "Data"=→"AI":waveform(dbl)[], "X Data"=w398:waveform(dbl)[], "AI stream data"=w383:dbl[][], "Y Data"=w397:waveform(dbl)[], "SUM Data"=w396:waveform(dbl)[])  [unwired: 4 in]
    n199 = case shown="True" "Data transfer method" {
      tunnel: w398 -> [_ w456]
      tunnel: w397 -> [_ w452]
      tunnel: w396 -> [_ w451]
      frame False {
      }
      frame True {
        n200 = call-poly <vilib>:"FFT Power Spectrum and PSD.vi"("time signals"=w456) -> ("Power Spectrum / PSD"=→"X PSD":cluster{"f0":dbl, "df":dbl, "magnitude":dbl[]}[])  [unwired: 7 in, 3 out]
        n201 = call-poly <vilib>:"FFT Power Spectrum and PSD.vi"("time signals"=w452) -> ("Power Spectrum / PSD"=→"Y PSD":cluster{"f0":dbl, "df":dbl, "magnitude":dbl[]}[])  [unwired: 7 in, 3 out]
        n202 = call-poly <vilib>:"FFT Power Spectrum and PSD.vi"("time signals"=w451) -> ("Power Spectrum / PSD"=→"SUM PSD":cluster{"f0":dbl, "df":dbl, "magnitude":dbl[]}[])  [unwired: 7 in, 3 out]
        "X" <- w456
        "Y" <- w452
        "SUM" <- w451
      }
    }
    n203 = call "check_folder.vi"("path in"="Save Path Directory") -> ("path out"=w388:path)
    n204 = case shown="True" "Save data" {
      tunnel: w388 -> [_ w441]
      tunnel: "File name" -> [_ w440]
      tunnel: w386 -> [_ w439]
      tunnel: w385 -> [_ w438]
      tunnel: w384 -> [_ w437]
      tunnel: w383 -> [_ w436]
      tunnel: w382 -> [_ w435]
      tunnel: w381 -> [_ w434]
      tunnel: "Data transfer method" -> [_ w433]
      frame False {
      }
      frame True {
        n205 = call "save_data.vi"("AI stream data"=w436, "Beam sorted SUM data"=w437, "Beam sorted Y data"=w438, "Beam sorted X data"=w439, "Collection type"=w433, "File name"=w440, "Save Path Directory"=w441, "AI stream sampling rate"=w434, "Beam sorted sampling rate"=w435) -> ()
      }
    }
    n206 = in-place {
      in-place-border: [w464] -> w428
      in-place-border: w418 -> [w466]
      n207 = in-place-dvr #13(w427) -> (w465:bool, w463:errorcluster)
      n208 = Compound Arithmetic op=OR(w466, w465, w463) -> (w464:bool)
      n209 = in-place-dvr #13(w464) -> ()  [unwired: 2 out]
    }
    n210 = Wait (ms)(milliseconds to wait=u32 200) -> ()  [unwired: 1 out]
  }
  n211 = Merge Errors(w10, w9) -> (w11:errorcluster)
  n212 = xnode "Read/Write Control"("FPGA VI Reference In"=w17, "error in"=w11, "stream.request state 2"=3) -> ("FPGA VI Reference Out"=w14:refnum<k20>, "error out"=w16:errorcluster)
  n213 = xnode "Close FPGA VI Reference"("FPGA VI Reference In"=w14, "error in"=w16) -> ("error out"=w24:errorcluster)
  n214 = call <vilib>:"Simple Error Handler.vi"("error in (no error)"=w24) -> ("error out"=→"Error Out":errorcluster)  [unwired: 4 in, 4 out]
